vi "get Polynom and EPA Auswahl from SPAN and Comp Index.vi"(10 "Component Index":i32, 11 "SPAN Idx":i32) -> (0 "Index Cluster":T3, 2 "EPA Optionsfeld out":T1, 3 "Polynom-Ordnung out":T2)   [LabVIEW 2020, in "Linearisierung v2.lvlib" / "Gasteiler.lvlib"]
uses:
  Gasteiler/Gasteiler.lvlib
  Auswahl Polynom Ordnung.ctl
  EPA Optionsfeld.ctl
  Protokoll/Protokoll.lvlib
  Linearisierung v2.lvlib
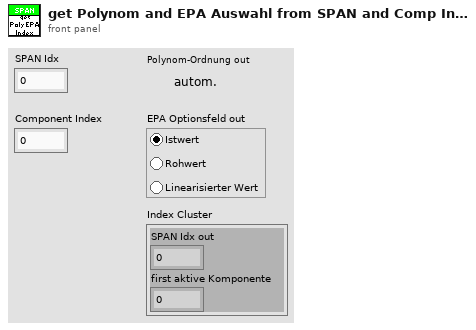
[diagram p1: front panel]
types:
  T1 = typedef "Linearisierung v2.lvlib/EPA Optionsfeld.ctl" = enum32{"Istwert", "Rohwert", "Linearisierter Wert"}
  T2 = typedef "Linearisierung v2.lvlib/Auswahl Polynom Ordnung.ctl" = enum16{"autom.", "raw", "actual", "1", "2", "3", "4"}
  T3 = cluster{"SPAN Idx out":i32, "first aktive Komponente":i32}
  T4 = typedef "Linearisierung v2.lvlib/Protokoll.lvlib/Aktion LIN Polynom Ordnung je Komponente für Protokoll.ctl" = enum16{"lesen", "schreiben", "init", "schreiben viewonly", "init initial"}
  T5 = typedef "Linearisierung v2.lvlib/Protokoll.lvlib/Aktion EPA Polynom Ordnung je Komponente für Protokoll.ctl" = enum16{"lesen", "schreiben", "init", "init initial"}
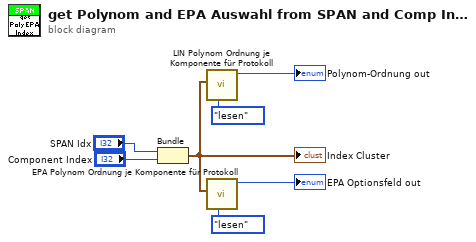
[diagram p0: block diagram]
diagram:
  n1 = Bundle("SPAN Idx"="SPAN Idx", "Component Index"="Component Index") -> (w7:cluster{"SPAN Idx":i32, "Component Index":i32})  [unwired: 1 in]
  "Index Cluster" <- w7
  n2 = call "LIN Polynom Ordnung je Komponente für Protokoll.vi"("Aktion"=Aktion_LIN_Polynom_Ordnung_je_Komponente_für_Protokoll."lesen", "Index in"=w7) -> ("Polynom-Ordnung out"=→"Polynom-Ordnung out":T2)  [unwired: 3 in, 6 out]
  n3 = call "EPA Polynom Ordnung je Komponente für Protokoll.vi"("Aktion"=Aktion_EPA_Polynom_Ordnung_je_Komponente_für_Protokoll."lesen", "Index in"=w7) -> ("EPA Optionsfeld out"=→"EPA Optionsfeld out":T1)  [unwired: 5 in, 3 out]
